vi "Test Dynamic Data.vi"() -> ()   [LabVIEW 2015]
uses:
  <vilib>/express/express shared/transition.llb/Dynamic To Waveform Array.vi
  <vilib>/express/express signal manip/GetorSetDDTAttributes/Set DDT Attributes/SetT0.vi
  <vilib>/express/express shared/transition.llb/Waveform Array To Dynamic.vi
  <vilib>/express/express signal manip/GetorSetDDTAttributes/Set DDT Attributes/Set DDT Properties.xnode
panel:
  out "Waveform Graph":dbl[](graph)
  out "Array":timestamp[][](array[timestamp])
  in  "Names":string[](array[string])=["CH1", "chan 2", "Bdot"]
  in  "Array - Numeric":cdb[](array[numeric])=[10.0+116.0i, 17.0+384.0i, -3.0-240.0i]
  in  "File Path Control":path=path "C:/Data/test.tdms"
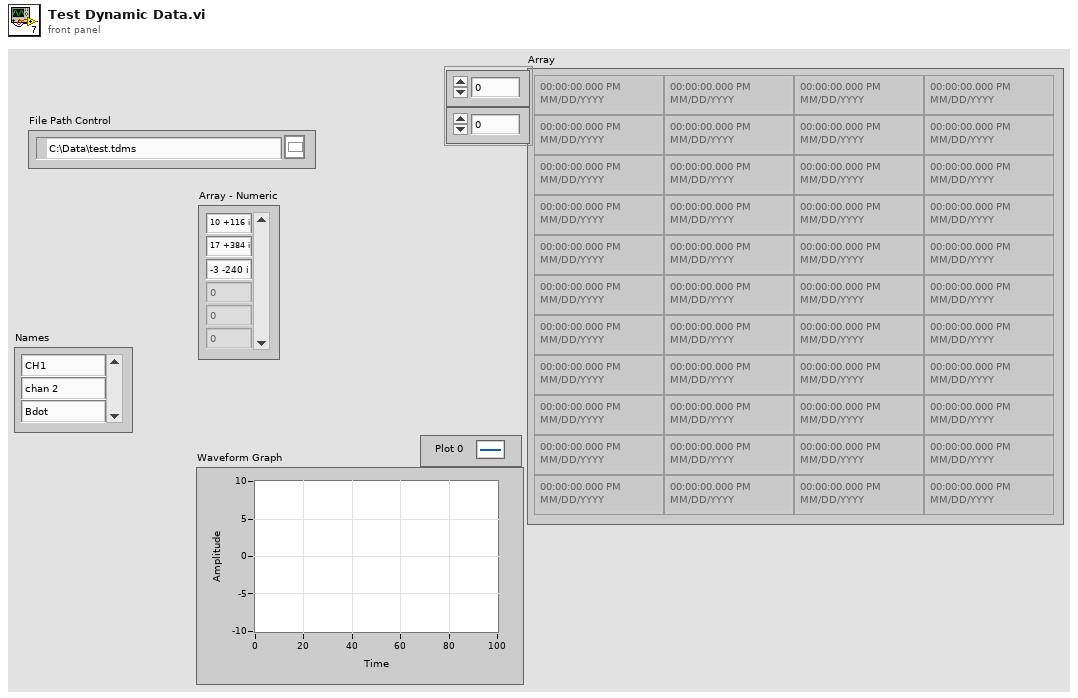
[diagram p1: front panel]
types:
  T1 = enum16{"open", "open or create", "create or replace", "create", "open (read-only)"}
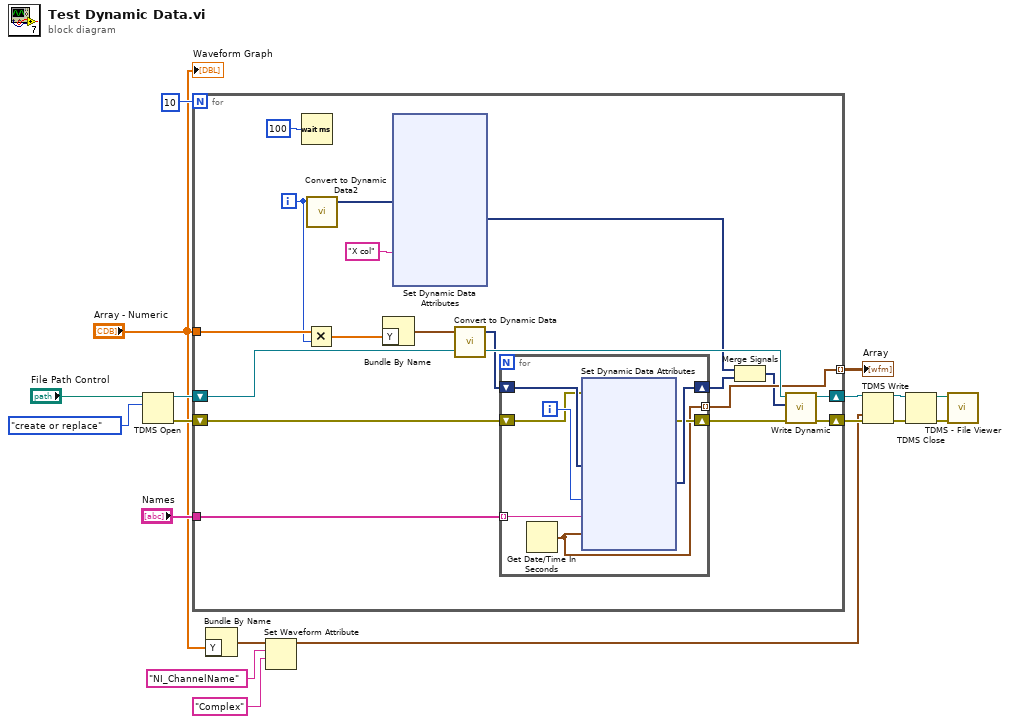
[diagram p0: block diagram]
diagram:
  n1 = TDMS Open(10:T1."create or replace" ("operation (0:open)"), 11:"File Path Control") -> (0:w11:errorcluster, 3:w16:refnum<k34>)  [unwired: 5 in]
  n2 = for {
    N: 10 -> [_]
    tunnel: "Array - Numeric" -> [w29]
    tunnel: "Names" -> [w33]
    shift-right: [w34] -> w15
    shift-left: w16 -> [w36]
    shift-right: [w35] -> w6
    shift-left: w11 -> [w32]
    tunnel: [w28] -> w9 mode=indexing
    i -> [w27]
    n3 = Wait (ms)(milliseconds to wait=u32 100) -> ()  [unwired: 1 out]
    n4 = Multiply(x=w29, y=w27) -> (x*y=w20:cdb[])
    n5 = call "Convert to Dynamic Data2"("Double"=w27) -> ("Dynamic Data Type"=w25:dynamicdata)  [unwired: 3 in]
    n6 = Bundle By Name("Y"=w20) -> (w19:waveform(cdb))  [unwired: 1 in]
    n7 = xnode "Set Dynamic Data Attributes"("Signals In"=w25, "Signal Name"="X col") -> ("Signals Out"=w24:dynamicdata)  [unwired: 3 in, 1 out]
    n8 = call "Convert to Dynamic Data"("Waveform"=w19) -> ("Dynamic Data Type"=w26:dynamicdata)  [unwired: 3 in]
    n9 = for {
      tunnel: w33 -> [w59] mode=indexing
      shift-right: [w58] -> w22
      shift-left: w26 -> [w61]
      shift-right: [w56] -> w31
      shift-left: w32 -> [w57]
      tunnel: [w55] -> w28 mode=indexing
      i -> [w60]
      n10 = Get Date/Time In Seconds() -> (seconds since 1Jan1904=w55:timestamp)
      n11 = xnode "Set Dynamic Data Attributes"("Signals In"=w61, "Signal Index"=w60, "Signal Name"=w59, "Timestamp"=w55, "error in"=w57) -> ("Signals Out"=w58:dynamicdata, "error out"=w56:errorcluster)
    }
    n12 = Merge Signals(w24, w22) -> (w21:dynamicdata)
    n13 = call "Write Dynamic.vi"("error in (no error)"=w31, "Dynamic data"=w21, "tdms file"=w36) -> ("error out"=w35:errorcluster, "tdms file out"=w34:refnum<k34>)  [unwired: 7 in]
  }
  "Array" <- w9
  n14 = Bundle By Name("Y"="Array - Numeric") -> (w4:waveform(cdb))  [unwired: 1 in]
  n15 = Set Waveform Attribute(5:"Complex" ("name"), 6:"NI_ChannelName" ("name"), 7:w4) -> (3:w3:waveform(cdb))  [unwired: 1 in, 2 out]
  n16 = TDMS Write(0:w15, 9:w3, 11:w6) -> (4:w8:refnum<k34>, 15:w7:errorcluster)  [unwired: 3 in, 2 out]
  n17 = TDMS Close(8:w7, 11:w8) -> (0:w14:errorcluster, 3:w13:path)
  n18 = call <vilib>:"TDMS - File Viewer.vi"("error in (no error)"=w14, "file path"=w13) -> ()  [unwired: 4 in, 2 out]
  "Waveform Graph" <- "Array - Numeric"
